vi "Read ImData.vi"(8 "error in (no error)":errorcluster, 10 "ReadSize":u32, 11 "AODAcq in":refnum<class "AODAcq.lvclass">) -> (0 "error out":errorcluster, 2 "ImData":waveform(i32)[](array[waveform]), 3 "AODAcq out":refnum<class "AODAcq.lvclass">)   [LabVIEW 2011, in "AODAcq.lvclass"]
uses:
  AODAcq.lvclass
  AODAcq.lvclass/AODAcq.ctl
  <instrlib>/niHWS/nihws.llb/niHWS Set Wfm DBL Attribute ID.ctl
  <vilib>/Utility/error.llb/Error Cluster From Error Code.vi
  <vilib>/rvi/errors/niLvFpgaAdjustHostInterfaceError.vi
  <instrlib>/niHWS/nihws.llb/niHWS Write Analog I32.vi
  <vilib>/rvi/interface/nirviMethod/nirviMethod.xnode
  FPGA_Control/AODRef.ctl
  FPGA_Control/FPGA Bitfiles/AODControl_FPGATarget_5751Acquire_F1CF9257.lvbitx
  FPGA_Control/AOD Control (FPGA).vi
  <vilib>/FPGAPlugInAG/PXIe-7965R/niLvFpga_ReadFifo_PXIe-7965R.vi
  <vilib>/rvi/errors/niLvFpgaMergeErrorWithErrorCode.vi
panel:
  out "Samples":i32
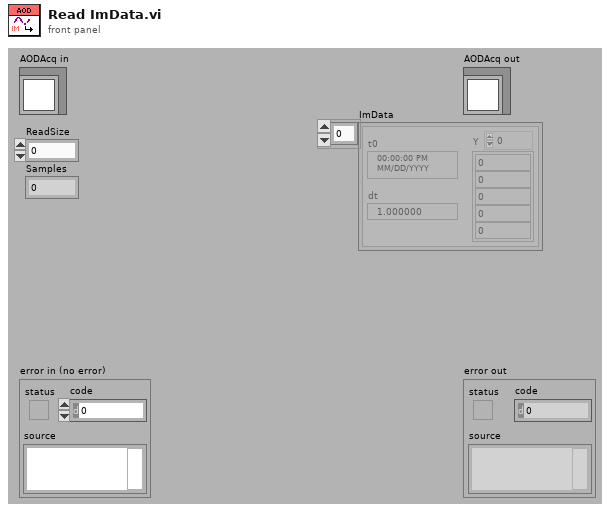
[diagram p1: front panel]
types:
  T1 = typedef "AODRef.ctl" = refnum<k20>
  T2 = typedef "niHWS Set Wfm DBL Attribute ID.ctl" = u32
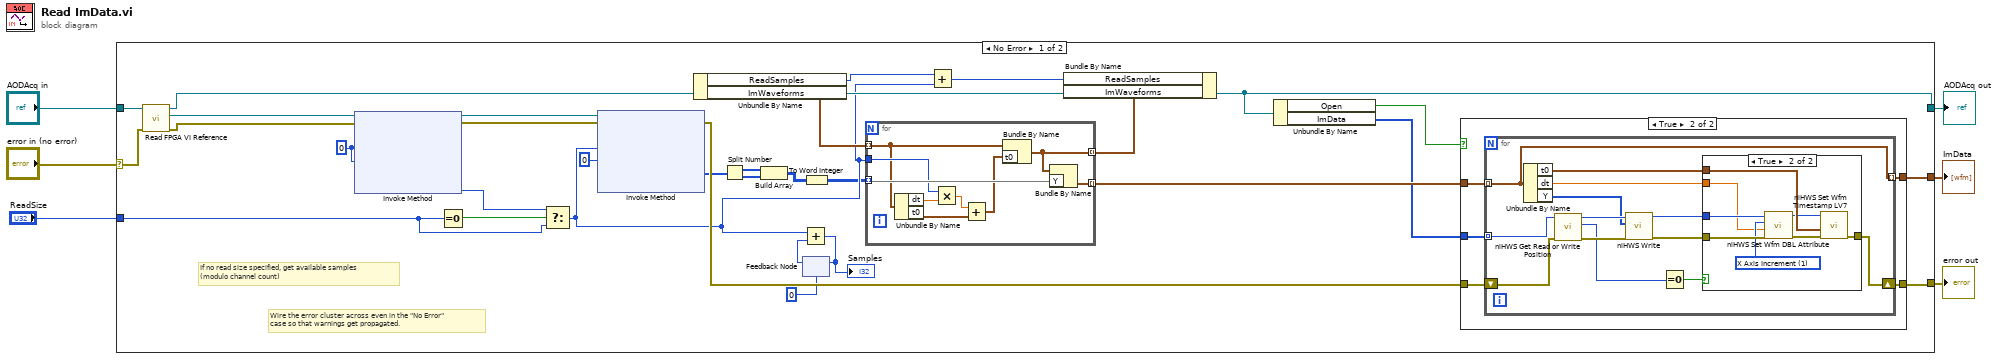
[diagram p0: block diagram]
diagram:
  n1 = case shown="No Error" "error in (no error)" {
    selector: "error in (no error)" -> [w32 w78]
    tunnel: [w23 w78] -> w5
    tunnel: [w27 w77] -> w3
    tunnel: "AODAcq in" -> [w38 w77]
    tunnel: "ReadSize" -> [w16 _]
    tunnel: [w22 _] -> w1
    frame No Error {
      w37 = u32 0 ("Number of Elements")
      # "If no read size specified, get available samples \n(modulo channel count)"
      # "Wire the error cluster across even in the \"No Error\"\ncase so that warnings get propagated."
      n2 = call-dynamic "Read FPGA VI Reference.vi"("error in (no error)"=w32, "AODAcq in"=w38) -> ("error out"=w9:errorcluster, "FPGA VI Reference"=w10:T1, "AODAcq out"=w30:refnum<class "AODAcq.lvclass">)  [unwired: 7 in]
      n3 = xnode "Invoke Method"("FPGA VI Reference In"=w10, "error in"=w9, "Number of Elements"=w37, "Timeout (ms)"=w37) -> ("FPGA VI Reference Out"=w35:T1, "error out"=w34:errorcluster, "Elements Remaining"=w12:u32)  [unwired: 1 out]
      n4 = Equal To 0?(x=w16) -> (x = 0?=w36:bool)
      n5 = Select(t=w12, s=w36, f=w16) -> (s? t:f=w13:u32)
      n6 = xnode "Invoke Method"("FPGA VI Reference In"=w35, "error in"=w34, "Number of Elements"=w13, "Timeout (ms)"=0) -> ("error out"=w24:errorcluster, "Data"=w15:i32[])  [unwired: 2 out]
      n7 = Unbundle By Name(w30) -> ("ReadSamples"=w21:u64, "ImWaveforms"=w31:waveform(i32)[])
      n8 = Split Number(x=w15) -> (hi(x)=w8:u16[], lo(x)=w7:u16[])
      n9 = Build Array(w8, w7) -> (w14:u16[][])
      n10 = feedback #1(0) -> (w18:u32)
      n11 = Add(x=w13, y=w18) -> (x+y=w19:u32)
      "Samples" <- w19
      n12 = feedback-in #1(w19) -> ()
      n13 = To Word Integer(number=w14) -> (16bit integer=w11:i16[][])
      n14 = for {
        tunnel: w11 -> [w76] mode=indexing
        tunnel: [w75] -> w28 mode=indexing
        tunnel: w31 -> [w70] mode=indexing
        tunnel: w13 -> [w73]
        tunnel: [w68] -> w29 mode=indexing
        n15 = Unbundle By Name(w70) -> ("dt"=w74:dbl, "t0"=w71:timestamp)
        n16 = Multiply(x=w73, y=w74) -> (x*y=w72:dbl)
        n17 = Add(x=w72, y=w71) -> (x+y=w69:timestamp)
        n18 = Bundle By Name(cluster=w70, "t0"=w69) -> (w68:waveform(i32))
        n19 = Bundle By Name(cluster=w68, "Y"=w76) -> (w75:waveform(i32))
      }
      n20 = Add(x=w21, y=w13) -> (x+y=w20:u64)
      n21 = Bundle By Name(cluster=w30, "ReadSamples"=w20, "ImWaveforms"=w29) -> (w27:refnum<class "AODAcq.lvclass">)
      n22 = Unbundle By Name(w27) -> ("Open"=w26:bool, "ImData"=w25:u32[])
      n23 = case shown="True" w26 {
        tunnel: w28 -> [w39 w45]
        tunnel: w25 -> [_ w44]
        tunnel: w24 -> [w40 w43]
        tunnel: [w40 w42] -> w23
        tunnel: [w39 w41] -> w22
        frame False {
        }
        frame True {
          n24 = for {
            tunnel: w45 -> [w46] mode=indexing
            tunnel: w44 -> [w50] mode=indexing
            shift-right: [w47] -> w42
            shift-left: w43 -> [w52]
            tunnel: [w46] -> w41 mode=indexing
            n25 = Unbundle By Name(w46) -> ("t0"=w48:timestamp, "dt"=w49:dbl, "Y"=w51:i32[])
            n26 = call <instrlib>:"niHWS Get Read or Write Position.vi"("waveform reference in"=w50, "error in (no error)"=w52) -> ("waveform reference out"=w57:u32, "position"=w54:u32, "error out"=w56:errorcluster)  [unwired: 6 out]
            n27 = call-poly <instrlib>:"niHWS Write.vi"("error in (no error)"=w56, "data"=w51, "waveform reference in"=w57) -> ("error out"=w55:errorcluster, "waveform reference out"=w58:u32)  [unwired: 7 in]
            n28 = Equal To 0?(x=w54) -> (x = 0?=w53:bool)
            n29 = case shown="True" w53 {
              tunnel: w48 -> [_ w66]
              tunnel: [w59 w65] -> w47
              tunnel: w55 -> [w59 w63]
              tunnel: w58 -> [_ w62]
              tunnel: w49 -> [_ w60]
              frame False {
              }
              frame True {
                w61 = T2 1 items=["X Axis Start"=0, "X Axis Increment"=1, "Y Axis Minimum"=3, "Y Axis Maximum"=4] ("Attribute ID")
                n30 = call <instrlib>:"niHWS Set Wfm DBL Attribute.vi"("error in (no error)"=w63, "attribute value"=w60, "attribute ID"=w61, "waveform reference in"=w62) -> ("error out"=w67:errorcluster, "waveform reference out"=w64:u32)  [unwired: 6 out]
                n31 = call <instrlib>:"niHWS Set Wfm Timestamp LV7.vi"("error in (no error)"=w67, "waveform timestamp"=w66, "waveform reference in"=w64) -> ("error out"=w65:errorcluster)  [unwired: 8 out]
              }
            }
          }
        }
      }
    }
    frame Error {
    }
  }
  "error out" <- w5
  "AODAcq out" <- w3
  "ImData" <- w1
